vi "Chroma 1905x Series 488.2 Qry -SRE-.vi"(8 "error in (no error)":errorcluster, 11 "VISA resource name":refnum<visa-resource-name>) -> (0 "error out":errorcluster, 2 "Result":string, 3 "VISA resource name out":refnum<visa-resource-name>)   [LabVIEW 2025]
panel:
  # "*SRE?"
  # "Service Request Enable query"
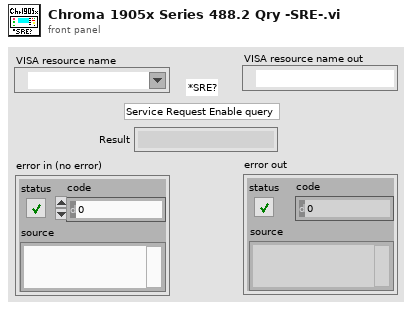
[diagram p1: front panel]
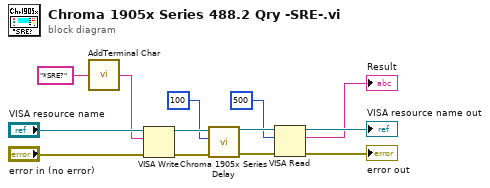
[diagram p0: block diagram]
diagram:
  n1 = call "AddTerminal Char.vi"("Cmd string"="*SRE?") -> ("Concatenated String"=w3:string)  [unwired: 4 in]
  n2 = VISA Write(VISA resource name="VISA resource name", write buffer=w3, error in (no error)="error in (no error)") -> (VISA resource name out=w9:refnum<visa-resource-name>, error out=w8:errorcluster)  [unwired: 1 out]
  n3 = call "Chroma 1905x Series Delay.vi"("error in (no error)"=w8, "Time Delay [ms]"=u32 100 ("Time Delay S"), "VISA resource name"=w9) -> ("error out"=w12:errorcluster, "VISA resource name 2"=w11:refnum<visa-resource-name>)  [unwired: 7 in]
  n4 = VISA Read(VISA resource name=w11, byte count=u32 500 ("byte count (0)"), error in (no error)=w12) -> (VISA resource name out=→"VISA resource name out":refnum<visa-resource-name>, read buffer=→"Result":string, error out=→"error out":errorcluster)  [unwired: 1 out]
